vi "Datasocket(多个信号)服务器.vi"() -> ()   [LabVIEW 2017]
uses:
  <vilib>/Analysis/NI_AALBase.lvlib
  <vilib>/measure/NI_MABase.lvlib
panel:
  in  "amplitude":dbl=1.0 caption="幅值" format="%0.2f"
  out "波形图 2":waveform(dbl)(graph)
  out "波形图":dbl[](graph)
  in  "停止":bool
  in  "frequency":dbl=10.0 caption="频率" format="%0.2p"
  in  "signal type":T1(ring) caption="信号类型"
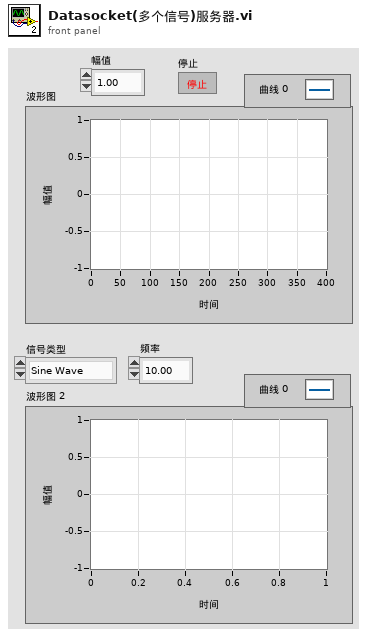
[diagram p1: front panel]
types:
  T1 = enum16{"Sine Wave", "Triangle Wave", "Square Wave", "Sawtooth Wave"}
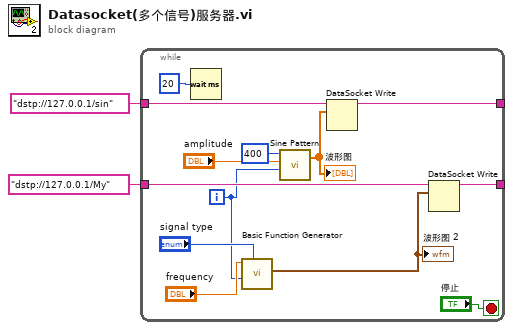
[diagram p0: block diagram]
diagram:
  n1 = while {
    tunnel: "dstp://127.0.0.1/sin" ("连接输入") -> [w15]
    tunnel: "dstp://127.0.0.1/My" ("连接输入") -> [w14]
    tunnel: [w9] -> _
    tunnel: [w8] -> _
    i -> [w3]
    stop <- "停止" stop-if-true
    n2 = Wait (ms)(milliseconds to wait=u32 20 ("等待时间（毫秒）")) -> ()  [unwired: 1 out]
    n3 = call <vilib>:"Basic Function Generator.vi"("signal type"="signal type", "phase"=w3, "frequency"="frequency") -> ("signal out"=w5:waveform(dbl))  [unwired: 6 in, 2 out]
    "波形图 2" <- w5
    n4 = call <vilib>:"Sine Pattern.vi"("phase(degrees)"=w3, "amplitude"="amplitude", "samples"=400) -> ("Sinusoidal Pattern"=w6:dbl[])  [unwired: 1 in, 1 out]
    "波形图" <- w6
    n5 = DataSocket Write(10:w6, 11:w15) -> (3:w9:string)  [unwired: 2 in, 2 out]
    n6 = DataSocket Write(10:w5, 11:w14) -> (3:w8:string)  [unwired: 2 in, 2 out]
  }
